vi "FTW-File-TextRead.vi"(0 "Filepath":path, 5 "Create if doesn't exist?":bool, 11 "error in":errorcluster) -> (4 "Filepath out":path, 6 "Text":string, 15 "error out":errorcluster)   [LabVIEW 2014]
panel:
  # "Inputs"
  # "Outputs"
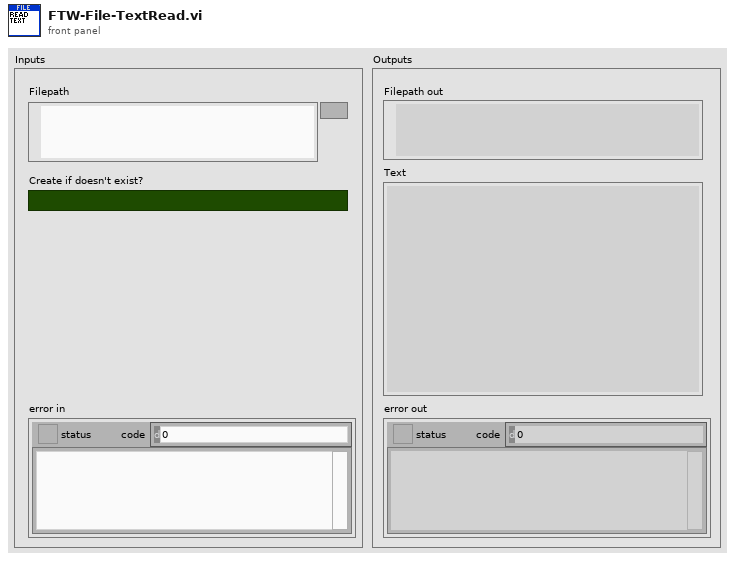
[diagram p1: front panel]
types:
  T1 = enum16{"open", "replace", "create", "open or create", "replace or create", "replace or create with confirmation"}
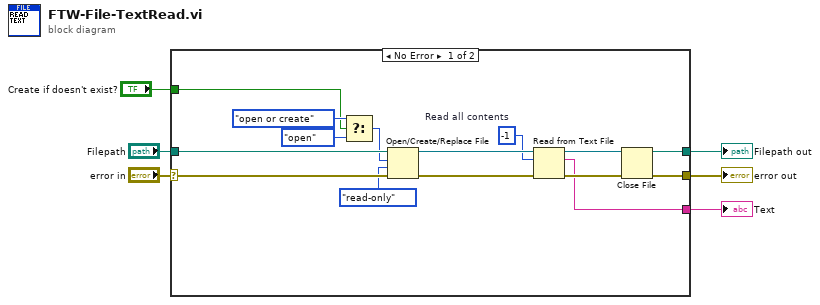
[diagram p0: block diagram]
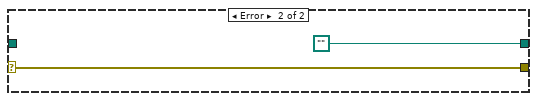
[diagram p2: hidden frame]
diagram:
  n1 = case shown="No Error" "error in" {
    selector: "error in" -> [w14 w22]
    tunnel: "Filepath" -> [w17 _]
    tunnel: [w16 path ""] -> w5
    tunnel: [w15 w22] -> w4
    tunnel: [w12 _] -> w2
    tunnel: "Create if doesn't exist?" -> [w8 _]
    frame No Error {
      w11 = -1  # Read all contents
      n2 = Select(t=T1."open or create" ("operation (0:open)"), s=w8, f=T1."open" ("operation (0:open)")) -> (s? t:f=w7:T1)
      n3 = Open/Create/Replace File(file path (use dialog)=w17, error in=w14, operation (0:open)=w7, access (0:read/write)=enum16{"read/write", "read-only", "write-only"}."read-only") -> (refnum out=w18:refnum<file>, error out=w19:errorcluster)  [unwired: 2 in, 1 out]
      n4 = Read from Text File(file (use dialog)=w18, count=w11, error in=w19) -> (refnum out=w21:refnum<file>, text=w12:string, error out=w20:errorcluster)  [unwired: 1 in, 1 out]
      n5 = Close File(refnum=w21, error in=w20) -> (path=w16:path, error out=w15:errorcluster)
    }
    frame Error {
    }
  }
  "error out" <- w4
  "Filepath out" <- w5
  "Text" <- w2
